vi "DCCH-Demo.vi"   [LabVIEW 2020]
panel:
  # "Run Me! :-)\n\n(More fun if the 24 VDC is on)\n\nThen check out the diagram"
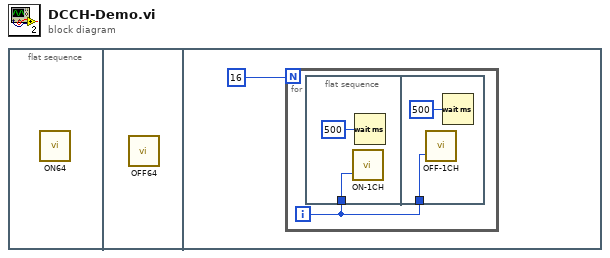
[diagram p0: block diagram]
diagram:
  n1 = flat-sequence {
    frame #0 {
      n2 = call "ON64.vi"() -> ()  [unwired: 1 in, 1 out]
    }
    frame #1 {
      n3 = call "OFF64.vi"() -> ()  [unwired: 1 in, 1 out]
    }
    frame #2 {
      n4 = for {
        N: 16 -> [_]
        i -> [w2]
        n5 = flat-sequence {
          tunnel: w2 -> [w4]
          tunnel: w2 -> [w6]
          frame #0 {
            n6 = call "ON-1CH.vi"("CH(0-63)"=w4) -> ()  [unwired: 1 in, 1 out]
            n7 = Wait (ms)(milliseconds to wait=u32 500) -> ()  [unwired: 1 out]
          }
          frame #1 {
            n8 = call "OFF-1CH.vi"("CH(0-63)"=w6) -> ()  [unwired: 1 in, 1 out]
            n9 = Wait (ms)(milliseconds to wait=u32 500) -> ()  [unwired: 1 out]
          }
        }
      }
    }
  }
